vi "Turn To Angle Teleop.vi"(8 "Z Axis":dbl, 9 "PID gains":T1={"proportional gain (Kc)"=0.035, "integral time (Ti, min)"=0.0, "derivative time (Td, min)"=0.0018}, 10 "POV":i16(knob) scale=0.0..360.0, 11 "output range":cluster{"output high":dbl, "output low":dbl}={"output high"=1.0, "output low"=-1.0}) -> (2 "Adjustment Voltage":dbl)   [LabVIEW 2018]
uses:
  <vilib>/addons/control/pid/pid.llb/PID (DBL).vi
  <vilib>/addons/control/pid/NI_PID_pid.lvlib
panel:
  # ".0202"
  # "0"
  # ".0032150"
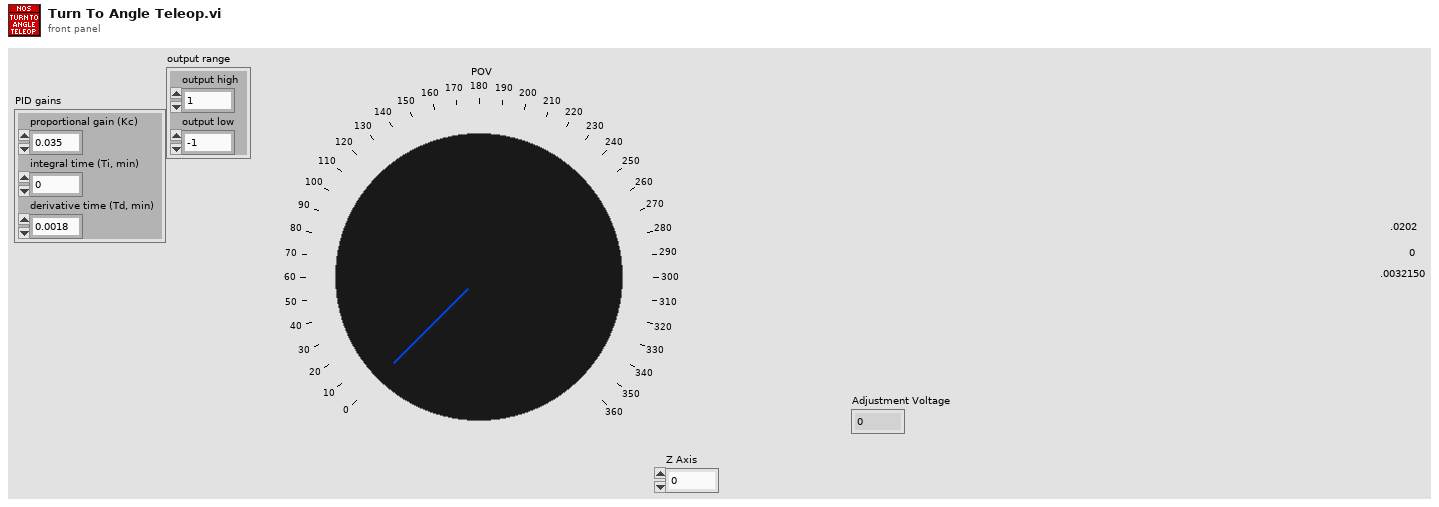
[diagram p1: front panel]
types:
  T1 = cluster{"proportional gain (Kc)":dbl, "integral time (Ti, min)":dbl, "derivative time (Td, min)":dbl}
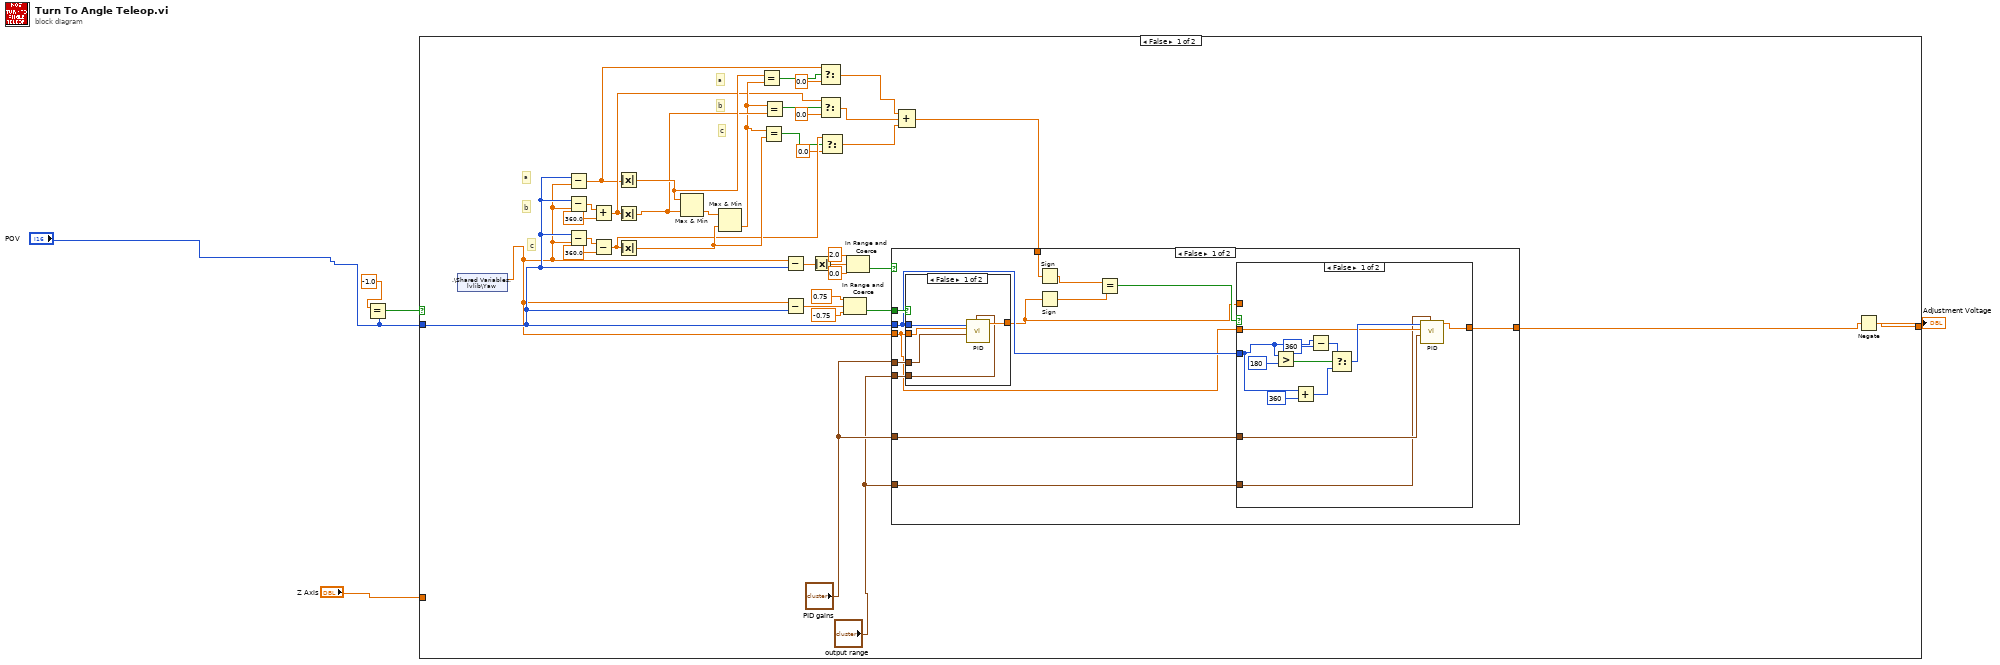
[diagram p0: block diagram]
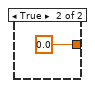
[diagram p3: hidden frame]
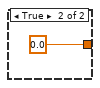
[diagram p4: hidden frame]
diagram:
  n1 = Equal?(x=-1.0, y="POV") -> (x = y?=w1:bool)
  n2 = case shown="False" w1 {
    tunnel: "POV" -> [w11 _]
    tunnel: [w12 w76] -> w4
    tunnel: "Z Axis" -> [_ w76]
    frame False {
      # "c"
      # "b"
      # "a"
      # "c"
      # "b"
      # "a"
      n3 = shared-variable ".\\Shared Variables.lvlib\\Yaw"() -> (w6:dbl)  [unwired: 1 in, 1 out]
      n4 = Subtract(x=w11, y=w6) -> (x-y=w22:dbl)
      n5 = Subtract(x=w11, y=w6) -> (x-y=w33:dbl)
      n6 = Subtract(x=w11, y=w6) -> (x-y=w31:dbl)
      n7 = Add(x=w33, y=360.0) -> (x+y=w23:dbl)
      n8 = Subtract(x=w31, y=360.0) -> (x-y=w21:dbl)
      n9 = Absolute Value(x=w22) -> (abs(x)=w28:dbl)
      n10 = Absolute Value(x=w23) -> (abs(x)=w27:dbl)
      n11 = Absolute Value(x=w21) -> (abs(x)=w25:dbl)
      n12 = Max & Min(x=w28, y=w27) -> (min(x,y)=w29:dbl)  [unwired: 1 out]
      n13 = Max & Min(x=w29, y=w25) -> (min(x,y)=w26:dbl)  [unwired: 1 out]
      n14 = Equal?(x=w28, y=w26) -> (x = y?=w20:bool)
      n15 = Equal?(x=w26, y=w25) -> (x = y?=w19:bool)
      n16 = Equal?(x=w26, y=w27) -> (x = y?=w24:bool)
      n17 = Subtract(x=w6, y=w11) -> (x-y=w40:dbl)
      n18 = Subtract(x=w6, y=w11) -> (x-y=w38:dbl)
      n19 = Absolute Value(x=w40) -> (abs(x)=w39:dbl)
      n20 = Select(t=w22, s=w20, f=0.0) -> (s? t:f=w15:dbl)
      n21 = Select(t=w23, s=w24, f=0.0) -> (s? t:f=w14:dbl)
      n22 = Select(t=w21, s=w19, f=0.0) -> (s? t:f=w13:dbl)
      n23 = In Range and Coerce(upper limit=0.75, x=w38, lower limit=-0.75) -> (In Range?=w35:bool)  [unwired: 1 out]
      n24 = In Range and Coerce(upper limit=2.0, x=w39, lower limit=0.0) -> (In Range?=w34:bool)  [unwired: 1 out]
      n25 = Compound Arithmetic op=ADD(w15, w14, w13) -> (w10:dbl)
      n26 = case shown="False" w34 {
        tunnel: w6 -> [w46 _]
        tunnel: w35 -> [w55 _]
        tunnel: w11 -> [w47 _]
        tunnel: "PID gains" -> [w54 _]
        tunnel: "output range" -> [w53 _]
        tunnel: w10 -> [w50 _]
        tunnel: [w49 0.0 ("output")] -> w9
        tunnel: "PID gains" -> [w45 _]
        tunnel: "output range" -> [w44 _]
        frame False {
          n27 = case shown="False" w55 {
            tunnel: w46 -> [w73 _]
            tunnel: w47 -> [w71 _]
            tunnel: [w72 0.0 ("output")] -> w43
            tunnel: w54 -> [w70 _]
            tunnel: w53 -> [w69 _]
            frame False {
              n28 = call-poly <vilib>:"PID.vi"("output range"=w69, "PID gains"=w70, "process variable"=w73, "setpoint"=w71) -> ("output"=w72:dbl)  [unwired: 6 in, 1 out]
            }
            frame True {
            }
          }
          n29 = Sign(1:w50) -> (0:w51:dbl)
          n30 = Sign(1:w43) -> (0:w52:dbl)
          n31 = Equal?(x=w51, y=w52) -> (x = y?=w48:bool)
          n32 = case shown="False" w48 {
            tunnel: [w67 w68] -> w49
            tunnel: w47 -> [w59 _]
            tunnel: w46 -> [w58 _]
            tunnel: w45 -> [w57 _]
            tunnel: w44 -> [w56 _]
            tunnel: w43 -> [_ w68]
            frame False {
              n33 = Greater?(x=w59, y=i16 180) -> (0:w65:bool)
              n34 = Add(x=w59, y=i16 360) -> (x+y=w63:i16)
              n35 = Subtract(x=w59, y=i16 360) -> (x-y=w61:i16)
              n36 = Select(t=w61, s=w65, f=w63) -> (s? t:f=w60:i16)
              n37 = call-poly <vilib>:"PID.vi"("output range"=w56, "PID gains"=w57, "process variable"=w58, "setpoint"=w60) -> ("output"=w67:dbl)  [unwired: 6 in, 1 out]
            }
            frame True {
            }
          }
        }
        frame True {
        }
      }
      n38 = Negate(x=w9) -> (-x=w12:dbl)
    }
    frame True {
    }
  }
  "Adjustment Voltage" <- w4
